vi "Reset.vi"(8 "error in (no error)":errorcluster caption="entrée d'erreur (pas d'erreur)", 11 "Class Spectrum_Analyser RS306B en entrée":refnum<class "Class Spectrum_Analyser RS306B.lvclass">) -> (0 "error out":errorcluster caption="sortie d'erreur", 3 "Class Spectrum_Analyser RS306B en sortie":refnum<class "Class Spectrum_Analyser RS306B.lvclass">)   [LabVIEW 2020, in "Library Instrument & Equipement.lvlib" / "Library Spectrum Analyser.lvlib" / "Class Spectrum_Analyser RS306B.lvclass"]
uses:
  Class Spectrum_Analyser RS306B.lvclass
  Class Spectrum Analyser (Default)/Class Spectrum Analyser (Default).lvclass
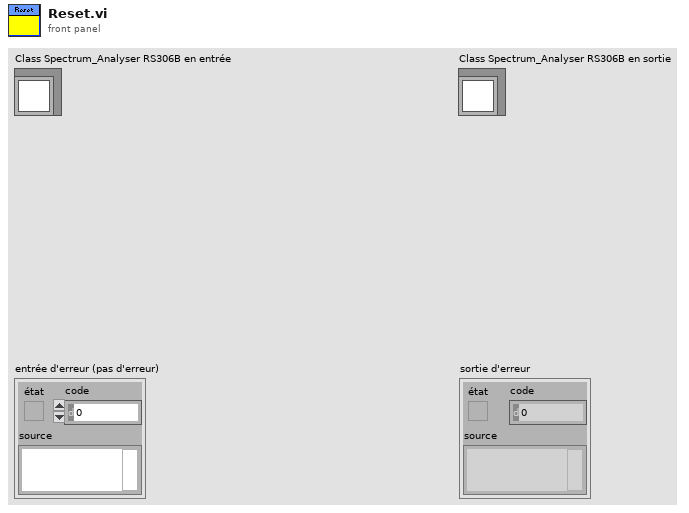
[diagram p1: front panel]
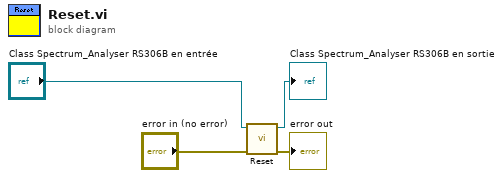
[diagram p0: block diagram]
diagram:
  n1 = call-parent "Reset.vi"("error in (no error)"="error in (no error)", "Class Spectrum Analyser (Default) en entrée"="Class Spectrum_Analyser RS306B en entrée") -> ("error out"=→"error out":errorcluster, "Class Spectrum Analyser (Default) en sortie"=→"Class Spectrum_Analyser RS306B en sortie":refnum<class "Class Spectrum_Analyser RS306B.lvclass">)  [unwired: 8 in]
